vi "Load App.vi"(8 "error in (no error)":errorcluster, 11 "Status Notifier":refnum<notifier>) -> (0 "error out":errorcluster)   [LabVIEW 2012, in "Actor Template.lvlib" / "Actor Template.lvclass"]
doc: "Load the application into memory and start it running. The input notifier is used to send text to the splash screen to tell the user what stage the load process is in."
uses:
  Actor Template.lvclass
  <vilib>/ActorFramework/Message Queue/Message Queue.lvclass/Message Queue.ctl
  <vilib>/ActorFramework/Actor/Actor.lvclass
  <vilib>/ActorFramework/Message Queue/Message Queue.lvclass
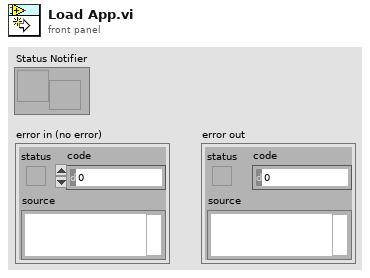
[diagram p1: front panel]
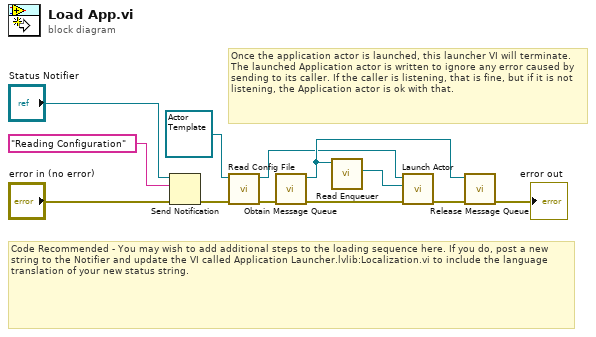
[diagram p0: block diagram]
diagram:
  # "Once the application actor is launched, this launcher VI will terminate. The launched Application actor is written to ignore any error caused by sending to its caller. If the caller is listening, that is fine, but if it is not listening, the Application actor is ok with that."
  # "Code Recommended - You may wish to add additional steps to the loading sequence here. If you do, post a new string to the Notifier and update the VI called Application Launcher.lvlib:Localization.vi to include the language translation of your new status string."
  n1 = Send Notification(notification="Reading Configuration", notifier="Status Notifier", error in (no error)="error in (no error)") -> (error out=w8:errorcluster)  [unwired: 1 out]
  n2 = call-dynamic "Read Config File.vi"("error in (no error)"=w8, "Actor Template in"=refnum<class "Actor Template.lvclass"> refnum ("My Application.lvclass")) -> ("error out"=w4:errorcluster, "Actor Template out"=w1:refnum<class "Actor Template.lvclass">)  [unwired: 8 in]
  n3 = call <vilib>:"Obtain Message Queue.vi"("error in (no error)"=w4) -> ("error out"=w3:errorcluster, "Message Queue"=w2:refnum<class "Message Queue.lvclass">)  [unwired: 9 in]
  n4 = call <vilib>:"Read Enqueuer.vi"("Message Queue"=w2) -> ("Message Enqueuer"=w7:refnum<class "Message Enqueuer.lvclass">)  [unwired: 10 in]
  n5 = call <vilib>:"Launch Actor.vi"("error in (no error)"=w3, "Actor-to-Caller Enqueuer"=w7, "Actor"=w1) -> ("error out"=w6:errorcluster)  [unwired: 7 in, 1 out]
  n6 = call <vilib>:"Release Message Queue.vi"("error in (no error)"=w6, "Message Queue"=w2) -> ("error out"=→"error out":errorcluster)  [unwired: 8 in, 1 out]
